vi "Lab Panel V6.00.vi"() -> ()   [LabVIEW 2017] (continued)
                                n1144 = TDMS Open(6:FALSE, 10:T23."create or replace" ("operation (0:open)"), 11:w2143) -> (0:w2142:errorcluster, 3:→"TDMS LAB05-2":refnum<k34>)  [unwired: 4 in]
                              }
                              frame #2 {
                                n1145 = local read "SET LAB05-2"() -> (w2153:T5)
                                n1146 = local read "TDMS LAB05-2"() -> (w2164:refnum<k34>)
                                n1147 = Build Array("Testers Name", "Description", "Set Test Cycles", "T-Rise minutes", "T-Rise Deg C") -> (w2154:string[])
                                n1148 = Unbundle(w2153) -> ("NAME"=w2152:string, "DESCRIPTION"=w2151:string, "CYCLES"=w2150:dbl, "T-RISE mins"=w2149:dbl, "T-RISE deg C"=w2148:dbl)
                                n1149 = Number To Decimal String(number=w2150) -> (decimal integer string=w2163:string)  [unwired: 1 in]
                                n1150 = Number To Decimal String(number=w2149) -> (decimal integer string=w2162:string)  [unwired: 1 in]
                                n1151 = Number To Decimal String(number=w2148) -> (decimal integer string=w2161:string)  [unwired: 1 in]
                                n1152 = Build Array(w2152, w2151, w2163, w2162, w2161) -> (w2160:string[])
                                n1153 = TDMS Set Properties(5:w2160, 7:w2154, 11:w2164) -> ()  [unwired: 3 in, 4 out]
                              }
                              frame #3 {
                                n1154 = local read "DISP LAB05-2"() -> (w2169:T4)
                                n1155 = Concatenate Strings("LAB05-2  ", w2167) -> (w2170:string)
                                n1156 = Two Button Dialog(message=w2170, 1:w2165, 2:w2166) -> (T button?=w2172:bool)
                                n1157 = case shown="True" w2172 {
                                tunnel: w2169 -> [w2179 w2180]
                                tunnel: [w2179 w2180] -> w2176
                                tunnel: [w2178 w2181] -> w2175
                                tunnel: [w2177 w2181] -> w2174
                                frame False {
                                n1158 = Unbundle(w2179) -> ("CYCLE"=w2178:dbl, "MINS"=w2177:dbl)  [unwired: 1 out]
                                }
                                frame True {
                                w2181 = 0.0
                                }
                                }
                                n1159 = Bundle(cluster=w2176, "CYCLE"=w2175, "MINS"=w2174, "STATUS"="RUN") -> (w2168:T4)
                                n1160 = local write "DISP LAB05-2"(w2168) -> ()
                              }
                              frame #4 {
                                n1161 = local read "TEMP START LAB05-2"() -> (w2184:cluster{"TL":dbl, "TN":dbl})
                                n1162 = Bundle(cluster=w2184, "TL"=w2182, "TN"=w2182) -> (w2183:cluster{"TL":dbl, "TN":dbl})
                                n1163 = local write "TEMP START LAB05-2"(w2183) -> ()
                              }
                            }
                          }
                        }
                      }
                    }
                  }
                }
                n1164 = local write "run lab05-2"(w2049) -> ()
              }
            }
            n1165 = local write "data file error"(w753) -> ()
          }
          frame #5 {
            # "Check if test cycles reached for cycle tests, if so then test pass"
            n1166 = stacked-sequence {
              tunnel: w2204 -> [_ _ _ _ _ _ _ _ _ _]
              tunnel: w2203 -> [_ _ _ _ _ _ _ _ _ _]
              tunnel: w2202 -> [_ _ _ _ _ _ _ _ _ _]
              tunnel: w2201 -> [_ _ _ _ _ _ _ _ _ _]
              tunnel: w2200 -> [_ _ _ _ _ _ _ _ _ _]
              tunnel: w2199 -> [_ _ _ _ _ _ _ _ _ _]
              tunnel: w2198 -> [_ _ _ _ _ _ _ _ _ _]
              tunnel: w2197 -> [_ _ _ _ _ _ _ _ _ _]
              tunnel: w2196 -> [_ _ _ _ _ _ _ _ _ _]
              tunnel: w2195 -> [_ _ _ _ _ _ _ _ _ _]
              tunnel: w2194 -> [w2210 _ _ _ _ _ _ _ _ _]
              tunnel: w2193 -> [_ w2245 _ _ _ _ _ _ _ _]
              tunnel: w2192 -> [_ _ w2285 _ _ _ _ _ _ _]
              tunnel: w2191 -> [_ _ _ w2325 _ _ _ _ _ _]
              tunnel: w2190 -> [_ _ _ _ w2365 _ _ _ _ _]
              tunnel: w2189 -> [_ _ _ _ _ w2405 _ _ _ _]
              tunnel: w2188 -> [_ _ _ _ _ _ w2445 _ _ _]
              tunnel: w2187 -> [_ _ _ _ _ _ _ w2485 _ _]
              tunnel: w2186 -> [_ _ _ _ _ _ _ _ w2525 _]
              tunnel: w2185 -> [_ _ _ _ _ _ _ _ _ w2565]
              frame #0 {
                # "LAB01-1"
                n1167 = Less?(x=w2210, y=2) -> (x < y?=w2208:bool)
                n1168 = local read "DISP LAB01-1"() -> (w2211:T4)
                n1169 = Unbundle By Name(w2211) -> ("STATUS"=w2205:string)
                n1170 = Equal?(x=w2205, y="RUN") -> (x = y?=w2207:bool)
                n1171 = And(x=w2207, y=w2208) -> (x .and. y?=w2206:bool)
                n1172 = case shown="True" w2206 {
                  tunnel: w2211 -> [_ w2216]
                  tunnel: w2210 -> [_ w2220]
                  frame False {
                  }
                  frame True {
                    n1173 = local read "SET LAB01-1"() -> (w2222:T5)
                    n1174 = local read "TDMS LAB01-1"() -> (w2215:refnum<k34>)
                    n1175 = Unbundle(w2222) -> ("CYCLES"=w2213:dbl, "T-RISE mins"=w2219:dbl)  [unwired: 3 out]
                    n1176 = case shown="\"CYCLE TEST\"" w2220 {
                      tunnel: w2219 -> [_ _ w2229]
                      tunnel: [w2224 w2226 w2229] -> w2218
                      tunnel: w2213 -> [w2224 w2226 _]
                      tunnel: ["CHART PASS" "CYCLE PASS" "T-RISE PASS"] -> w2217
                      frame "CHART TEST", Default {
                      }
                      frame "CYCLE TEST" {
                      }
                      frame "T-RISE TEST" {
                      }
                    }
                    n1177 = Unbundle(w2216) -> ("CYCLE"=w2221:dbl)  [unwired: 2 out]
                    n1178 = Increment(x=w2213) -> (x+1=w2214:dbl)
                    n1179 = Greater Or Equal?(x=w2221, y=w2214) -> (x >= y?=w2223:bool)
                    n1180 = case shown="True" w2223 {
                      tunnel: w2218 -> [w2233 _]
                      tunnel: w2217 -> [w2232 _]
                      tunnel: w2216 -> [w2231 _]
                      tunnel: w2215 -> [w2230 _]
                      frame True {
                        n1181 = stacked-sequence {
                          tunnel: w2233 -> [w2237 _]
                          tunnel: w2232 -> [w2235 w2241]
                          tunnel: w2231 -> [_ w2244]
                          tunnel: w2230 -> [w2234 _]
                          frame #0 {
                            n1182 = Build Array(w2235) -> (w2238:string[])
                            n1183 = Build Array(w2237) -> (w2236:dbl[])
                            n1184 = TDMS Write(0:w2234, 5:"TEST PASS", 7:w2238, 9:w2236) -> (15:w2240:errorcluster)  [unwired: 2 in, 3 out]
                            n1185 = local write "data file error"(w2240) -> ()
                          }
                          frame #1 {
                            n1186 = Bundle(cluster=w2244, "STATUS"=w2241) -> (w2242:T4)  [unwired: 2 in]
                            n1187 = local write "RESULT LAB01-1"(TRUE) -> ()
                            n1188 = local write "DISP LAB01-1"(w2242) -> ()
                          }
                        }
                      }
                      frame False {
                      }
                    }
                  }
                }
              }
              frame #1 {
                # "LAB01-2"
                n1189 = Less?(x=w2245, y=2) -> (x < y?=w2248:bool)
                n1190 = local read "DISP LAB01-2"() -> (w2250:T4)
                n1191 = Unbundle(w2250) -> ("STATUS"=w2251:string)  [unwired: 2 out]
                n1192 = Equal?(x=w2251, y="RUN") -> (x = y?=w2247:bool)
                n1193 = And(x=w2247, y=w2248) -> (x .and. y?=w2246:bool)
                n1194 = case shown="True" w2246 {
                  tunnel: w2250 -> [_ w2256]
                  tunnel: w2245 -> [_ w2260]
                  frame False {
                  }
                  frame True {
                    n1195 = local read "SET LAB01-2"() -> (w2262:T5)
                    n1196 = local read "TDMS LAB01-2"() -> (w2255:refnum<k34>)
                    n1197 = Unbundle(w2262) -> ("CYCLES"=w2253:dbl, "T-RISE mins"=w2259:dbl)  [unwired: 3 out]
                    n1198 = case shown="\"T-RISE TEST\"" w2260 {
                      tunnel: w2259 -> [_ _ w2269]
                      tunnel: [w2264 w2266 w2269] -> w2258
                      tunnel: w2253 -> [w2264 w2266 _]
                      tunnel: ["CHART PASS" "CYCLE PASS" "T-RISE PASS"] -> w2257
                      frame "CHART TEST", Default {
                      }
                      frame "CYCLE TEST" {
                      }
                      frame "T-RISE TEST" {
                      }
                    }
                    n1199 = Unbundle(w2256) -> ("CYCLE"=w2261:dbl)  [unwired: 2 out]
                    n1200 = Increment(x=w2253) -> (x+1=w2254:dbl)
                    n1201 = Greater Or Equal?(x=w2261, y=w2254) -> (x >= y?=w2263:bool)
                    n1202 = case shown="True" w2263 {
                      tunnel: w2258 -> [w2273 _]
                      tunnel: w2257 -> [w2272 _]
                      tunnel: w2256 -> [w2271 _]
                      tunnel: w2255 -> [w2270 _]
                      frame True {
                        n1203 = stacked-sequence {
                          tunnel: w2273 -> [w2277 _]
                          tunnel: w2272 -> [w2275 w2281]
                          tunnel: w2271 -> [_ w2284]
                          tunnel: w2270 -> [w2274 _]
                          frame #0 {
                            n1204 = Build Array(w2275) -> (w2278:string[])
                            n1205 = Build Array(w2277) -> (w2276:dbl[])
                            n1206 = TDMS Write(0:w2274, 5:"TEST PASS", 7:w2278, 9:w2276) -> (15:w2280:errorcluster)  [unwired: 2 in, 3 out]
                            n1207 = local write "data file error"(w2280) -> ()
                          }
                          frame #1 {
                            n1208 = Bundle(cluster=w2284, "STATUS"=w2281) -> (w2282:T4)  [unwired: 2 in]
                            n1209 = local write "RESULT LAB01-2"(TRUE) -> ()
                            n1210 = local write "DISP LAB01-2"(w2282) -> ()
                          }
                        }
                      }
                      frame False {
                      }
                    }
                  }
                }
              }
              frame #2 {
                # "LAB02-1"
                n1211 = Less?(x=w2285, y=2) -> (x < y?=w2288:bool)
                n1212 = local read "DISP LAB02-1"() -> (w2290:T4)
                n1213 = Unbundle(w2290) -> ("STATUS"=w2291:string)  [unwired: 2 out]
                n1214 = Equal?(x=w2291, y="RUN") -> (x = y?=w2287:bool)
                n1215 = And(x=w2287, y=w2288) -> (x .and. y?=w2286:bool)
                n1216 = case shown="True" w2286 {
                  tunnel: w2290 -> [_ w2296]
                  tunnel: w2285 -> [_ w2300]
                  frame False {
                  }
                  frame True {
                    n1217 = local read "TDMS LAB02-1"() -> (w2295:refnum<k34>)
                    n1218 = local read "SET LAB02-1"() -> (w2302:T5)
                    n1219 = Unbundle(w2296) -> ("CYCLE"=w2301:dbl)  [unwired: 2 out]
                    n1220 = Unbundle(w2302) -> ("CYCLES"=w2293:dbl, "T-RISE mins"=w2299:dbl)  [unwired: 3 out]
                    n1221 = case shown="\"T-RISE TEST\"" w2300 {
                      tunnel: w2299 -> [_ _ w2309]
                      tunnel: [w2304 w2306 w2309] -> w2298
                      tunnel: w2293 -> [w2304 w2306 _]
                      tunnel: ["CHART PASS" "CYCLE PASS" "T-RISE PASS"] -> w2297
                      frame "CHART TEST", Default {
                      }
                      frame "CYCLE TEST" {
                      }
                      frame "T-RISE TEST" {
                      }
                    }
                    n1222 = Increment(x=w2293) -> (x+1=w2294:dbl)
                    n1223 = Greater Or Equal?(x=w2301, y=w2294) -> (x >= y?=w2303:bool)
                    n1224 = case shown="True" w2303 {
                      tunnel: w2298 -> [w2313 _]
                      tunnel: w2297 -> [w2312 _]
                      tunnel: w2296 -> [w2311 _]
                      tunnel: w2295 -> [w2310 _]
                      frame True {
                        n1225 = stacked-sequence {
                          tunnel: w2313 -> [w2317 _]
                          tunnel: w2312 -> [w2315 w2321]
                          tunnel: w2311 -> [_ w2324]
                          tunnel: w2310 -> [w2314 _]
                          frame #0 {
                            n1226 = Build Array(w2315) -> (w2318:string[])
                            n1227 = Build Array(w2317) -> (w2316:dbl[])
                            n1228 = TDMS Write(0:w2314, 5:"TEST PASS", 7:w2318, 9:w2316) -> (15:w2320:errorcluster)  [unwired: 2 in, 3 out]
                            n1229 = local write "data file error"(w2320) -> ()
                          }
                          frame #1 {
                            n1230 = Bundle(cluster=w2324, "STATUS"=w2321) -> (w2322:T4)  [unwired: 2 in]
                            n1231 = local write "RESULT LAB02-1"(TRUE) -> ()
                            n1232 = local write "DISP LAB02-1"(w2322) -> ()
                          }
                        }
                      }
                      frame False {
                      }
                    }
                  }
                }
              }
              frame #3 {
                # "LAB02-2"
                n1233 = Less?(x=w2325, y=2) -> (x < y?=w2328:bool)
                n1234 = local read "DISP LAB02-2"() -> (w2330:T4)
                n1235 = Unbundle(w2330) -> ("STATUS"=w2331:string)  [unwired: 2 out]
                n1236 = Equal?(x=w2331, y="RUN") -> (x = y?=w2327:bool)
                n1237 = And(x=w2327, y=w2328) -> (x .and. y?=w2326:bool)
                n1238 = case shown="True" w2326 {
                  tunnel: w2330 -> [_ w2336]
                  tunnel: w2325 -> [_ w2340]
                  frame False {
                  }
                  frame True {
                    n1239 = local read "TDMS LAB02-2"() -> (w2335:refnum<k34>)
                    n1240 = local read "SET LAB02-2"() -> (w2342:T5)
                    n1241 = Unbundle(w2336) -> ("CYCLE"=w2341:dbl)  [unwired: 2 out]
                    n1242 = Unbundle(w2342) -> ("CYCLES"=w2333:dbl, "T-RISE mins"=w2339:dbl)  [unwired: 3 out]
                    n1243 = case shown="\"T-RISE TEST\"" w2340 {
                      tunnel: w2339 -> [_ _ w2349]
                      tunnel: [w2344 w2346 w2349] -> w2338
                      tunnel: w2333 -> [w2344 w2346 _]
                      tunnel: ["CHART PASS" "CYCLE PASS" "T-RISE PASS"] -> w2337
                      frame "CHART TEST", Default {
                      }
                      frame "CYCLE TEST" {
                      }
                      frame "T-RISE TEST" {
                      }
                    }
                    n1244 = Increment(x=w2333) -> (x+1=w2334:dbl)
                    n1245 = Greater Or Equal?(x=w2341, y=w2334) -> (x >= y?=w2343:bool)
                    n1246 = case shown="True" w2343 {
                      tunnel: w2338 -> [w2353 _]
                      tunnel: w2337 -> [w2352 _]
                      tunnel: w2336 -> [w2351 _]
                      tunnel: w2335 -> [w2350 _]
                      frame True {
                        n1247 = stacked-sequence {
                          tunnel: w2353 -> [w2357 _]
                          tunnel: w2352 -> [w2355 w2361]
                          tunnel: w2351 -> [_ w2364]
                          tunnel: w2350 -> [w2354 _]
                          frame #0 {
                            n1248 = Build Array(w2355) -> (w2358:string[])
                            n1249 = Build Array(w2357) -> (w2356:dbl[])
                            n1250 = TDMS Write(0:w2354, 5:"TEST PASS", 7:w2358, 9:w2356) -> (15:w2360:errorcluster)  [unwired: 2 in, 3 out]
                            n1251 = local write "data file error"(w2360) -> ()
                          }
                          frame #1 {
                            n1252 = Bundle(cluster=w2364, "STATUS"=w2361) -> (w2362:T4)  [unwired: 2 in]
                            n1253 = local write "RESULT LAB02-2"(TRUE) -> ()
                            n1254 = local write "DISP LAB02-2"(w2362) -> ()
                          }
                        }
                      }
                      frame False {
                      }
                    }
                  }
                }
              }
              frame #4 {
                # "LAB03-1"
                n1255 = Less?(x=w2365, y=2) -> (x < y?=w2368:bool)
                n1256 = local read "DISP LAB03-1"() -> (w2370:T4)
                n1257 = Unbundle(w2370) -> ("STATUS"=w2371:string)  [unwired: 2 out]
                n1258 = Equal?(x=w2371, y="RUN") -> (x = y?=w2367:bool)
                n1259 = And(x=w2367, y=w2368) -> (x .and. y?=w2366:bool)
                n1260 = case shown="True" w2366 {
                  tunnel: w2370 -> [_ w2376]
                  tunnel: w2365 -> [_ w2380]
                  frame False {
                  }
                  frame True {
                    n1261 = local read "TDMS LAB03-1"() -> (w2375:refnum<k34>)
                    n1262 = local read "SET LAB03-1"() -> (w2382:T5)
                    n1263 = Unbundle(w2376) -> ("CYCLE"=w2381:dbl)  [unwired: 2 out]
                    n1264 = Unbundle(w2382) -> ("CYCLES"=w2373:dbl, "T-RISE mins"=w2379:dbl)  [unwired: 3 out]
                    n1265 = case shown="\"T-RISE TEST\"" w2380 {
                      tunnel: w2379 -> [_ _ w2389]
                      tunnel: [w2384 w2386 w2389] -> w2378
                      tunnel: w2373 -> [w2384 w2386 _]
                      tunnel: ["CHART PASS" "CYCLE PASS" "T-RISE PASS"] -> w2377
                      frame "CHART TEST", Default {
                      }
                      frame "CYCLE TEST" {
                      }
                      frame "T-RISE TEST" {
                      }
                    }
                    n1266 = Increment(x=w2373) -> (x+1=w2374:dbl)
                    n1267 = Greater Or Equal?(x=w2381, y=w2374) -> (x >= y?=w2383:bool)
                    n1268 = case shown="True" w2383 {
                      tunnel: w2378 -> [w2393 _]
                      tunnel: w2377 -> [w2392 _]
                      tunnel: w2376 -> [w2391 _]
                      tunnel: w2375 -> [w2390 _]
                      frame True {
                        n1269 = stacked-sequence {
                          tunnel: w2393 -> [w2397 _]
                          tunnel: w2392 -> [w2395 w2401]
                          tunnel: w2391 -> [_ w2404]
                          tunnel: w2390 -> [w2394 _]
                          frame #0 {
                            n1270 = Build Array(w2395) -> (w2398:string[])
                            n1271 = Build Array(w2397) -> (w2396:dbl[])
                            n1272 = TDMS Write(0:w2394, 5:"TEST PASS", 7:w2398, 9:w2396) -> (15:w2400:errorcluster)  [unwired: 2 in, 3 out]
                            n1273 = local write "data file error"(w2400) -> ()
                          }
                          frame #1 {
                            n1274 = Bundle(cluster=w2404, "STATUS"=w2401) -> (w2402:T4)  [unwired: 2 in]
                            n1275 = local write "RESULT LAB03-1"(TRUE) -> ()
                            n1276 = local write "DISP LAB03-1"(w2402) -> ()
                          }
                        }
                      }
                      frame False {
                      }
                    }
                  }
                }
              }
              frame #5 {
                # "LAB03-2"
                n1277 = Less?(x=w2405, y=2) -> (x < y?=w2408:bool)
                n1278 = local read "DISP LAB03-2"() -> (w2410:T4)
                n1279 = Unbundle(w2410) -> ("STATUS"=w2411:string)  [unwired: 2 out]
                n1280 = Equal?(x=w2411, y="RUN") -> (x = y?=w2407:bool)
                n1281 = And(x=w2407, y=w2408) -> (x .and. y?=w2406:bool)
                n1282 = case shown="True" w2406 {
                  tunnel: w2410 -> [_ w2416]
                  tunnel: w2405 -> [_ w2420]
                  frame False {
                  }
                  frame True {
                    n1283 = local read "TDMS LAB03-2"() -> (w2415:refnum<k34>)
                    n1284 = local read "SET LAB03-2"() -> (w2422:T5)
                    n1285 = Unbundle(w2416) -> ("CYCLE"=w2421:dbl)  [unwired: 2 out]
                    n1286 = Unbundle(w2422) -> ("CYCLES"=w2413:dbl, "T-RISE mins"=w2419:dbl)  [unwired: 3 out]
                    n1287 = case shown="\"T-RISE TEST\"" w2420 {
                      tunnel: w2419 -> [_ _ w2429]
                      tunnel: [w2424 w2426 w2429] -> w2418
                      tunnel: w2413 -> [w2424 w2426 _]
                      tunnel: ["CHART PASS" "CYCLE PASS" "T-RISE PASS"] -> w2417
                      frame "CHART TEST", Default {
                      }
                      frame "CYCLE TEST" {
                      }
                      frame "T-RISE TEST" {
                      }
                    }
                    n1288 = Increment(x=w2413) -> (x+1=w2414:dbl)
                    n1289 = Greater Or Equal?(x=w2421, y=w2414) -> (x >= y?=w2423:bool)
                    n1290 = case shown="True" w2423 {
                      tunnel: w2418 -> [w2433 _]
                      tunnel: w2417 -> [w2432 _]
                      tunnel: w2416 -> [w2431 _]
                      tunnel: w2415 -> [w2430 _]
                      frame True {
                        n1291 = stacked-sequence {
                          tunnel: w2433 -> [w2437 _]
                          tunnel: w2432 -> [w2435 w2441]
                          tunnel: w2431 -> [_ w2444]
                          tunnel: w2430 -> [w2434 _]
                          frame #0 {
                            n1292 = Build Array(w2435) -> (w2438:string[])
                            n1293 = Build Array(w2437) -> (w2436:dbl[])
                            n1294 = TDMS Write(0:w2434, 5:"TEST PASS", 7:w2438, 9:w2436) -> (15:w2440:errorcluster)  [unwired: 2 in, 3 out]
                            n1295 = local write "data file error"(w2440) -> ()
                          }
                          frame #1 {
                            n1296 = Bundle(cluster=w2444, "STATUS"=w2441) -> (w2442:T4)  [unwired: 2 in]
                            n1297 = local write "RESULT LAB03-2"(TRUE) -> ()
                            n1298 = local write "DISP LAB03-2"(w2442) -> ()
                          }
                        }
                      }
                      frame False {
                      }
                    }
                  }
                }
              }
              frame #6 {
                # "LAB04-1"
                n1299 = Less?(x=w2445, y=2) -> (x < y?=w2448:bool)
                n1300 = local read "DISP LAB04-1"() -> (w2450:T4)
                n1301 = Unbundle(w2450) -> ("STATUS"=w2451:string)  [unwired: 2 out]
                n1302 = Equal?(x=w2451, y="RUN") -> (x = y?=w2447:bool)
                n1303 = And(x=w2447, y=w2448) -> (x .and. y?=w2446:bool)
                n1304 = case shown="True" w2446 {
                  tunnel: w2450 -> [_ w2456]
                  tunnel: w2445 -> [_ w2460]
                  frame False {
                  }
                  frame True {
                    n1305 = local read "TDMS LAB04-1"() -> (w2455:refnum<k34>)
                    n1306 = local read "SET LAB04-1"() -> (w2462:T5)
                    n1307 = Unbundle(w2456) -> ("CYCLE"=w2461:dbl)  [unwired: 2 out]
                    n1308 = Unbundle(w2462) -> ("CYCLES"=w2453:dbl, "T-RISE mins"=w2459:dbl)  [unwired: 3 out]
                    n1309 = case shown="\"T-RISE TEST\"" w2460 {
                      tunnel: w2459 -> [_ _ w2469]
                      tunnel: [w2464 w2466 w2469] -> w2458
                      tunnel: w2453 -> [w2464 w2466 _]
                      tunnel: ["CHART PASS" "CYCLE PASS" "T-RISE PASS"] -> w2457
                      frame "CHART TEST", Default {
                      }
                      frame "CYCLE TEST" {
                      }
                      frame "T-RISE TEST" {
                      }
                    }
                    n1310 = Increment(x=w2453) -> (x+1=w2454:dbl)
                    n1311 = Greater Or Equal?(x=w2461, y=w2454) -> (x >= y?=w2463:bool)
                    n1312 = case shown="True" w2463 {
                      tunnel: w2458 -> [w2473 _]
                      tunnel: w2457 -> [w2472 _]
                      tunnel: w2456 -> [w2471 _]
                      tunnel: w2455 -> [w2470 _]
                      frame True {
                        n1313 = stacked-sequence {
                          tunnel: w2473 -> [w2477 _]
                          tunnel: w2472 -> [w2475 w2481]
                          tunnel: w2471 -> [_ w2484]
                          tunnel: w2470 -> [w2474 _]
                          frame #0 {
                            n1314 = Build Array(w2475) -> (w2478:string[])
                            n1315 = Build Array(w2477) -> (w2476:dbl[])
                            n1316 = TDMS Write(0:w2474, 5:"TEST PASS", 7:w2478, 9:w2476) -> (15:w2480:errorcluster)  [unwired: 2 in, 3 out]
                            n1317 = local write "data file error"(w2480) -> ()
                          }
                          frame #1 {
                            n1318 = Bundle(cluster=w2484, "STATUS"=w2481) -> (w2482:T4)  [unwired: 2 in]
                            n1319 = local write "RESULT LAB04-1"(TRUE) -> ()
                            n1320 = local write "DISP LAB04-1"(w2482) -> ()
                          }
                        }
                      }
                      frame False {
                      }
                    }
                  }
                }
              }
              frame #7 {
                # "LAB04-2"
                n1321 = Less?(x=w2485, y=2) -> (x < y?=w2488:bool)
                n1322 = local read "DISP LAB04-2"() -> (w2490:T4)
                n1323 = Unbundle(w2490) -> ("STATUS"=w2491:string)  [unwired: 2 out]
                n1324 = Equal?(x=w2491, y="RUN") -> (x = y?=w2487:bool)
                n1325 = And(x=w2487, y=w2488) -> (x .and. y?=w2486:bool)
                n1326 = case shown="True" w2486 {
                  tunnel: w2490 -> [_ w2496]
                  tunnel: w2485 -> [_ w2500]
                  frame False {
                  }
                  frame True {
                    n1327 = local read "TDMS LAB04-2"() -> (w2495:refnum<k34>)
                    n1328 = local read "SET LAB04-2"() -> (w2502:T5)
                    n1329 = Unbundle(w2496) -> ("CYCLE"=w2501:dbl)  [unwired: 2 out]
                    n1330 = Unbundle(w2502) -> ("CYCLES"=w2493:dbl, "T-RISE mins"=w2499:dbl)  [unwired: 3 out]
                    n1331 = case shown="\"T-RISE TEST\"" w2500 {
                      tunnel: w2499 -> [_ _ w2509]
                      tunnel: [w2504 w2506 w2509] -> w2498
                      tunnel: w2493 -> [w2504 w2506 _]
                      tunnel: ["CHART PASS" "CYCLE PASS" "T-RISE PASS"] -> w2497
                      frame "CHART TEST", Default {
                      }
                      frame "CYCLE TEST" {
                      }
                      frame "T-RISE TEST" {
                      }
                    }
                    n1332 = Increment(x=w2493) -> (x+1=w2494:dbl)
                    n1333 = Greater Or Equal?(x=w2501, y=w2494) -> (x >= y?=w2503:bool)
                    n1334 = case shown="True" w2503 {
                      tunnel: w2498 -> [w2513 _]
                      tunnel: w2497 -> [w2512 _]
                      tunnel: w2496 -> [w2511 _]
                      tunnel: w2495 -> [w2510 _]
                      frame True {
                        n1335 = stacked-sequence {
                          tunnel: w2513 -> [w2517 _]
                          tunnel: w2512 -> [w2515 w2521]
                          tunnel: w2511 -> [_ w2524]
                          tunnel: w2510 -> [w2514 _]
                          frame #0 {
                            n1336 = Build Array(w2515) -> (w2518:string[])
                            n1337 = Build Array(w2517) -> (w2516:dbl[])
                            n1338 = TDMS Write(0:w2514, 5:"TEST PASS", 7:w2518, 9:w2516) -> (15:w2520:errorcluster)  [unwired: 2 in, 3 out]
                            n1339 = local write "data file error"(w2520) -> ()
                          }
                          frame #1 {
                            n1340 = Bundle(cluster=w2524, "STATUS"=w2521) -> (w2522:T4)  [unwired: 2 in]
                            n1341 = local write "RESULT LAB04-2"(TRUE) -> ()
                            n1342 = local write "DISP LAB04-2"(w2522) -> ()
                          }
                        }
                      }
                      frame False {
                      }
                    }
                  }
                }
              }
              frame #8 {
                # "LAB05-1"
                n1343 = Less?(x=w2525, y=2) -> (x < y?=w2528:bool)
                n1344 = local read "DISP LAB05-1"() -> (w2530:T4)
                n1345 = Unbundle(w2530) -> ("STATUS"=w2531:string)  [unwired: 2 out]
                n1346 = Equal?(x=w2531, y="RUN") -> (x = y?=w2527:bool)
                n1347 = And(x=w2527, y=w2528) -> (x .and. y?=w2526:bool)
                n1348 = case shown="True" w2526 {
                  tunnel: w2530 -> [_ w2536]
                  tunnel: w2525 -> [_ w2540]
                  frame False {
                  }
                  frame True {
                    n1349 = local read "TDMS LAB05-1"() -> (w2535:refnum<k34>)
                    n1350 = local read "SET LAB05-1"() -> (w2542:T5)
                    n1351 = Unbundle(w2536) -> ("CYCLE"=w2541:dbl)  [unwired: 2 out]
                    n1352 = Unbundle(w2542) -> ("CYCLES"=w2533:dbl, "T-RISE mins"=w2539:dbl)  [unwired: 3 out]
                    n1353 = case shown="\"T-RISE TEST\"" w2540 {
                      tunnel: w2539 -> [_ _ w2549]
                      tunnel: [w2544 w2546 w2549] -> w2538
                      tunnel: w2533 -> [w2544 w2546 _]
                      tunnel: ["CHART PASS" "CYCLE PASS" "T-RISE PASS"] -> w2537
                      frame "CHART TEST", Default {
                      }
                      frame "CYCLE TEST" {
                      }
                      frame "T-RISE TEST" {
                      }
                    }
                    n1354 = Increment(x=w2533) -> (x+1=w2534:dbl)
                    n1355 = Greater Or Equal?(x=w2541, y=w2534) -> (x >= y?=w2543:bool)
                    n1356 = case shown="True" w2543 {
                      tunnel: w2538 -> [w2553 _]
                      tunnel: w2537 -> [w2552 _]
                      tunnel: w2536 -> [w2551 _]
                      tunnel: w2535 -> [w2550 _]
                      frame True {
                        n1357 = stacked-sequence {
                          tunnel: w2553 -> [w2557 _]
                          tunnel: w2552 -> [w2555 w2561]
                          tunnel: w2551 -> [_ w2564]
                          tunnel: w2550 -> [w2554 _]
                          frame #0 {
                            n1358 = Build Array(w2555) -> (w2558:string[])
                            n1359 = Build Array(w2557) -> (w2556:dbl[])
                            n1360 = TDMS Write(0:w2554, 5:"TEST PASS", 7:w2558, 9:w2556) -> (15:w2560:errorcluster)  [unwired: 2 in, 3 out]
                            n1361 = local write "data file error"(w2560) -> ()
                          }
                          frame #1 {
                            n1362 = Bundle(cluster=w2564, "STATUS"=w2561) -> (w2562:T4)  [unwired: 2 in]
                            n1363 = local write "RESULT LAB05-1"(TRUE) -> ()
                            n1364 = local write "DISP LAB05-1"(w2562) -> ()
                          }
                        }
                      }
                      frame False {
                      }
                    }
                  }
                }
              }
              frame #9 {
                # "LAB05-2"
                n1365 = Less?(x=w2565, y=2) -> (x < y?=w2568:bool)
                n1366 = local read "DISP LAB05-2"() -> (w2570:T4)
                n1367 = Unbundle(w2570) -> ("STATUS"=w2571:string)  [unwired: 2 out]
                n1368 = Equal?(x=w2571, y="RUN") -> (x = y?=w2567:bool)
                n1369 = And(x=w2567, y=w2568) -> (x .and. y?=w2566:bool)
                n1370 = case shown="True" w2566 {
                  tunnel: w2570 -> [_ w2576]
                  tunnel: w2565 -> [_ w2580]
                  frame False {
                  }
                  frame True {
                    n1371 = local read "TDMS LAB05-2"() -> (w2575:refnum<k34>)
                    n1372 = local read "SET LAB05-2"() -> (w2582:T5)
                    n1373 = Unbundle(w2576) -> ("CYCLE"=w2581:dbl)  [unwired: 2 out]
                    n1374 = Unbundle(w2582) -> ("CYCLES"=w2573:dbl, "T-RISE mins"=w2579:dbl)  [unwired: 3 out]
                    n1375 = case shown="\"T-RISE TEST\"" w2580 {
                      tunnel: w2579 -> [_ _ w2589]
                      tunnel: [w2584 w2586 w2589] -> w2578
                      tunnel: w2573 -> [w2584 w2586 _]
                      tunnel: ["CHART PASS" "CYCLE PASS" "T-RISE PASS"] -> w2577
                      frame "CHART TEST", Default {
                      }
                      frame "CYCLE TEST" {
                      }
                      frame "T-RISE TEST" {
                      }
                    }
                    n1376 = Increment(x=w2573) -> (x+1=w2574:dbl)
                    n1377 = Greater Or Equal?(x=w2581, y=w2574) -> (x >= y?=w2583:bool)
                    n1378 = case shown="True" w2583 {
                      tunnel: w2578 -> [w2593 _]
                      tunnel: w2577 -> [w2592 _]
                      tunnel: w2576 -> [w2591 _]
                      tunnel: w2575 -> [w2590 _]
                      frame True {
                        n1379 = stacked-sequence {
                          tunnel: w2593 -> [w2597 _]
                          tunnel: w2592 -> [w2595 w2601]
                          tunnel: w2591 -> [_ w2604]
                          tunnel: w2590 -> [w2594 _]
                          frame #0 {
                            n1380 = Build Array(w2595) -> (w2598:string[])
                            n1381 = Build Array(w2597) -> (w2596:dbl[])
                            n1382 = TDMS Write(0:w2594, 5:"TEST PASS", 7:w2598, 9:w2596) -> (15:w2600:errorcluster)  [unwired: 2 in, 3 out]
                            n1383 = local write "data file error"(w2600) -> ()
                          }
                          frame #1 {
                            n1384 = Bundle(cluster=w2604, "STATUS"=w2601) -> (w2602:T4)  [unwired: 2 in]
                            n1385 = local write "RESULT LAB05-2"(TRUE) -> ()
                            n1386 = local write "DISP LAB05-2"(w2602) -> ()
                          }
                        }
                      }
                      frame False {
                      }
                    }
                  }
                }
              }
            }
          }
          frame #6 {
            # "check if test cycles reached for temperature rise test"
            n1387 = stacked-sequence {
              tunnel: w2634 -> [_ _ _ _ _ _ _ _ _ _]
              tunnel: w2633 -> [_ _ _ _ _ _ _ _ _ _]
              tunnel: w2632 -> [_ _ _ _ _ _ _ _ _ _]
              tunnel: w2631 -> [_ _ _ _ _ _ _ _ _ _]
              tunnel: w2630 -> [_ _ _ _ _ _ _ _ _ _]
              tunnel: w2629 -> [_ _ _ _ _ _ _ _ _ _]
              tunnel: w2628 -> [_ _ _ _ _ _ _ _ _ _]
              tunnel: w2627 -> [_ _ _ _ _ _ _ _ _ _]
              tunnel: w2626 -> [_ _ _ _ _ _ _ _ _ _]
              tunnel: w2625 -> [_ _ _ _ _ _ _ _ _ _]
              tunnel: w2624 -> [w2640 _ _ _ _ _ _ _ _ _]
              tunnel: w2614 -> [w2635 _ _ _ _ _ _ _ _ _]
              tunnel: w2623 -> [_ w2666 _ _ _ _ _ _ _ _]
              tunnel: w2622 -> [_ _ w2696 _ _ _ _ _ _ _]
              tunnel: w2621 -> [_ _ _ w2726 _ _ _ _ _ _]
              tunnel: w2620 -> [_ _ _ _ w2756 _ _ _ _ _]
              tunnel: w2619 -> [_ _ _ _ _ w2786 _ _ _ _]
              tunnel: w2618 -> [_ _ _ _ _ _ w2816 _ _ _]
              tunnel: w2617 -> [_ _ _ _ _ _ _ w2846 _ _]
              tunnel: w2616 -> [_ _ _ _ _ _ _ _ w2876 _]
              tunnel: w2615 -> [_ _ _ _ _ _ _ _ _ w2906]
              tunnel: w2613 -> [_ w2665 _ _ _ _ _ _ _ _]
              tunnel: w2612 -> [_ _ w2695 _ _ _ _ _ _ _]
              tunnel: w2611 -> [_ _ _ w2725 _ _ _ _ _ _]
              tunnel: w2610 -> [_ _ _ _ w2755 _ _ _ _ _]
              tunnel: w2609 -> [_ _ _ _ _ w2785 _ _ _ _]
              tunnel: w2608 -> [_ _ _ _ _ _ w2815 _ _ _]
              tunnel: w2607 -> [_ _ _ _ _ _ _ w2845 _ _]
              tunnel: w2606 -> [_ _ _ _ _ _ _ _ w2875 _]
              tunnel: w2605 -> [_ _ _ _ _ _ _ _ _ w2905]
              frame #0 {
                # "LAB01-1"
                n1388 = Equal?(x=w2640, y=2) -> (x = y?=w2638:bool)
                n1389 = local read "DISP LAB01-1"() -> (w2641:T4)
                n1390 = Unbundle By Name(w2641) -> ("STATUS"=w2642:string)
                n1391 = Equal?(x=w2642, y="RUN") -> (x = y?=w2637:bool)
                n1392 = And(x=w2637, y=w2638) -> (x .and. y?=w2636:bool)
                n1393 = case shown="True" w2636 {
                  tunnel: w2641 -> [_ w2645]
                  tunnel: w2635 -> [_ w2648]
                  frame False {
                  }
                  frame True {
                    n1394 = Unbundle By Name(w2645) -> ("CYCLE"=w2649:dbl)
                    n1395 = local read "SET LAB01-1"() -> (w2647:T5)
                    n1396 = local read "TDMS LAB01-1"() -> (w2644:refnum<k34>)
                    n1397 = Unbundle(w2647) -> ("T-RISE mins"=w2646:dbl)  [unwired: 4 out]
                    n1398 = Greater Or Equal?(x=w2649, y=w2648) -> (x >= y?=w2650:bool)
                    n1399 = case shown="True" w2650 {
                      tunnel: w2646 -> [w2653 _]
                      tunnel: w2645 -> [w2652 _]
                      tunnel: w2644 -> [w2651 _]
                      frame True {
                        n1400 = stacked-sequence {
                          tunnel: w2653 -> [w2656 _]
                          tunnel: w2652 -> [_ w2661]
                          tunnel: w2651 -> [w2654 _]
                          frame #0 {
                            n1401 = Build Array("T-RISE") -> (w2658:string[])
                            n1402 = Build Array(w2656) -> (w2657:dbl[])
                            n1403 = TDMS Write(0:w2654, 5:"TEST PASS", 7:w2658, 9:w2657) -> (15:w2660:errorcluster)  [unwired: 2 in, 3 out]
                            n1404 = local write "data file error"(w2660) -> ()
                          }
                          frame #1 {
                            n1405 = Bundle(cluster=w2661, "STATUS"="T-RISE PASS") -> (w2663:T4)  [unwired: 2 in]
                            n1406 = local write "RESULT LAB01-1"(TRUE) -> ()
                            n1407 = local write "DISP LAB01-1"(w2663) -> ()
                          }
                        }
                      }
                      frame False {
                      }
                    }
                  }
                }
              }
              frame #1 {
                # "LAB01-2"
                n1408 = Equal?(x=w2666, y=2) -> (x = y?=w2669:bool)
                n1409 = local read "DISP LAB01-2"() -> (w2671:T4)
                n1410 = Unbundle(w2671) -> ("STATUS"=w2672:string)  [unwired: 2 out]
                n1411 = Equal?(x=w2672, y="RUN") -> (x = y?=w2668:bool)
                n1412 = And(x=w2668, y=w2669) -> (x .and. y?=w2667:bool)
                n1413 = case shown="True" w2667 {
                  tunnel: w2671 -> [_ w2675]
                  tunnel: w2665 -> [_ w2678]
                  frame False {
                  }
                  frame True {
                    n1414 = local read "SET LAB01-2"() -> (w2677:T5)
                    n1415 = local read "TDMS LAB01-2"() -> (w2674:refnum<k34>)
                    n1416 = Unbundle(w2675) -> ("CYCLE"=w2679:dbl)  [unwired: 2 out]
                    n1417 = Unbundle(w2677) -> ("T-RISE mins"=w2676:dbl)  [unwired: 4 out]
                    n1418 = Greater Or Equal?(x=w2679, y=w2678) -> (x >= y?=w2680:bool)
                    n1419 = case shown="True" w2680 {
                      tunnel: w2676 -> [w2683 _]
                      tunnel: w2675 -> [w2682 _]
                      tunnel: w2674 -> [w2681 _]
                      frame True {
                        n1420 = stacked-sequence {
                          tunnel: w2683 -> [w2686 _]
                          tunnel: w2682 -> [_ w2691]
                          tunnel: w2681 -> [w2684 _]
                          frame #0 {
                            n1421 = Build Array("T-RISE") -> (w2688:string[])
                            n1422 = Build Array(w2686) -> (w2687:dbl[])
                            n1423 = TDMS Write(0:w2684, 5:"TEST PASS", 7:w2688, 9:w2687) -> (15:w2690:errorcluster)  [unwired: 2 in, 3 out]
                            n1424 = local write "data file error"(w2690) -> ()
                          }
                          frame #1 {
                            n1425 = Bundle(cluster=w2691, "STATUS"="T-RISE PASS") -> (w2693:T4)  [unwired: 2 in]
                            n1426 = local write "RESULT LAB01-2"(TRUE) -> ()
                            n1427 = local write "DISP LAB01-2"(w2693) -> ()
                          }
                        }
                      }
                      frame False {
                      }
                    }
                  }
                }
              }
              frame #2 {
                # "LAB02-1"
                n1428 = Equal?(x=w2696, y=2) -> (x = y?=w2699:bool)
                n1429 = local read "DISP LAB02-1"() -> (w2701:T4)
                n1430 = Unbundle(w2701) -> ("STATUS"=w2702:string)  [unwired: 2 out]
                n1431 = Equal?(x=w2702, y="RUN") -> (x = y?=w2698:bool)
                n1432 = And(x=w2698, y=w2699) -> (x .and. y?=w2697:bool)
                n1433 = case shown="True" w2697 {
                  tunnel: w2701 -> [_ w2705]
                  tunnel: w2695 -> [_ w2708]
                  frame False {
                  }
                  frame True {
                    n1434 = local read "SET LAB02-1"() -> (w2707:T5)
                    n1435 = local read "TDMS LAB02-1"() -> (w2704:refnum<k34>)
                    n1436 = Unbundle(w2705) -> ("CYCLE"=w2709:dbl)  [unwired: 2 out]
                    n1437 = Unbundle(w2707) -> ("T-RISE mins"=w2706:dbl)  [unwired: 4 out]
                    n1438 = Greater Or Equal?(x=w2709, y=w2708) -> (x >= y?=w2710:bool)
                    n1439 = case shown="True" w2710 {
                      tunnel: w2706 -> [w2713 _]
                      tunnel: w2705 -> [w2712 _]
                      tunnel: w2704 -> [w2711 _]
                      frame True {
                        n1440 = stacked-sequence {
                          tunnel: w2713 -> [w2716 _]
                          tunnel: w2712 -> [_ w2721]
                          tunnel: w2711 -> [w2714 _]
                          frame #0 {
                            n1441 = Build Array("T-RISE") -> (w2718:string[])
                            n1442 = Build Array(w2716) -> (w2717:dbl[])
                            n1443 = TDMS Write(0:w2714, 5:"TEST PASS", 7:w2718, 9:w2717) -> (15:w2720:errorcluster)  [unwired: 2 in, 3 out]
                            n1444 = local write "data file error"(w2720) -> ()
                          }
                          frame #1 {
                            n1445 = Bundle(cluster=w2721, "STATUS"="T-RISE PASS") -> (w2723:T4)  [unwired: 2 in]
                            n1446 = local write "RESULT LAB02-1"(TRUE) -> ()
                            n1447 = local write "DISP LAB02-1"(w2723) -> ()
                          }
                        }
                      }
                      frame False {
                      }
                    }
                  }
                }
              }
              frame #3 {
                # "LAB02-2"
                n1448 = Equal?(x=w2726, y=2) -> (x = y?=w2729:bool)
                n1449 = local read "DISP LAB02-2"() -> (w2731:T4)
                n1450 = Unbundle(w2731) -> ("STATUS"=w2732:string)  [unwired: 2 out]
                n1451 = Equal?(x=w2732, y="RUN") -> (x = y?=w2728:bool)
                n1452 = And(x=w2728, y=w2729) -> (x .and. y?=w2727:bool)
                n1453 = case shown="True" w2727 {
                  tunnel: w2731 -> [_ w2735]
                  tunnel: w2725 -> [_ w2738]
                  frame False {
                  }
                  frame True {
                    n1454 = local read "SET LAB02-2"() -> (w2737:T5)
                    n1455 = local read "TDMS LAB02-2"() -> (w2734:refnum<k34>)
                    n1456 = Unbundle(w2735) -> ("CYCLE"=w2739:dbl)  [unwired: 2 out]
                    n1457 = Unbundle(w2737) -> ("T-RISE mins"=w2736:dbl)  [unwired: 4 out]
                    n1458 = Greater Or Equal?(x=w2739, y=w2738) -> (x >= y?=w2740:bool)
                    n1459 = case shown="True" w2740 {
                      tunnel: w2736 -> [w2743 _]
                      tunnel: w2735 -> [w2742 _]
                      tunnel: w2734 -> [w2741 _]
                      frame True {
                        n1460 = stacked-sequence {
                          tunnel: w2743 -> [w2746 _]
                          tunnel: w2742 -> [_ w2751]
                          tunnel: w2741 -> [w2744 _]
                          frame #0 {
                            n1461 = Build Array("T-RISE") -> (w2748:string[])
                            n1462 = Build Array(w2746) -> (w2747:dbl[])
                            n1463 = TDMS Write(0:w2744, 5:"TEST PASS", 7:w2748, 9:w2747) -> (15:w2750:errorcluster)  [unwired: 2 in, 3 out]
                            n1464 = local write "data file error"(w2750) -> ()
                          }
                          frame #1 {
                            n1465 = Bundle(cluster=w2751, "STATUS"="T-RISE PASS") -> (w2753:T4)  [unwired: 2 in]
                            n1466 = local write "RESULT LAB02-2"(TRUE) -> ()
                            n1467 = local write "DISP LAB02-2"(w2753) -> ()
                          }
                        }
                      }
                      frame False {
                      }
                    }
                  }
                }
              }
              frame #4 {
                # "LAB03-1"
                n1468 = Equal?(x=w2756, y=2) -> (x = y?=w2759:bool)
                n1469 = local read "DISP LAB03-1"() -> (w2761:T4)
                n1470 = Unbundle(w2761) -> ("STATUS"=w2762:string)  [unwired: 2 out]
                n1471 = Equal?(x=w2762, y="RUN") -> (x = y?=w2758:bool)
                n1472 = And(x=w2758, y=w2759) -> (x .and. y?=w2757:bool)
                n1473 = case shown="True" w2757 {
                  tunnel: w2761 -> [_ w2765]
                  tunnel: w2755 -> [_ w2768]
                  frame False {
                  }
                  frame True {
                    n1474 = local read "SET LAB03-1"() -> (w2767:T5)
                    n1475 = local read "TDMS LAB03-1"() -> (w2764:refnum<k34>)
                    n1476 = Unbundle(w2765) -> ("CYCLE"=w2769:dbl)  [unwired: 2 out]
                    n1477 = Unbundle(w2767) -> ("T-RISE mins"=w2766:dbl)  [unwired: 4 out]
                    n1478 = Greater Or Equal?(x=w2769, y=w2768) -> (x >= y?=w2770:bool)
                    n1479 = case shown="True" w2770 {
                      tunnel: w2766 -> [w2773 _]
                      tunnel: w2765 -> [w2772 _]
                      tunnel: w2764 -> [w2771 _]
                      frame True {
                        n1480 = stacked-sequence {
                          tunnel: w2773 -> [w2776 _]
                          tunnel: w2772 -> [_ w2781]
                          tunnel: w2771 -> [w2774 _]
                          frame #0 {
                            n1481 = Build Array("T-RISE") -> (w2778:string[])
                            n1482 = Build Array(w2776) -> (w2777:dbl[])
                            n1483 = TDMS Write(0:w2774, 5:"TEST PASS", 7:w2778, 9:w2777) -> (15:w2780:errorcluster)  [unwired: 2 in, 3 out]
                            n1484 = local write "data file error"(w2780) -> ()
                          }
                          frame #1 {
                            n1485 = Bundle(cluster=w2781, "STATUS"="T-RISE PASS") -> (w2783:T4)  [unwired: 2 in]
                            n1486 = local write "RESULT LAB03-1"(TRUE) -> ()
